vi "get Approach wfm.vi"(0 "reference in":refnum<class "Fcurve.lvclass">, 1 "Zeroed (wfms.array)":waveform(dbl)[](array[waveform]), 5 "error in (no error)":errorcluster) -> (14 "reference out":refnum<class "Fcurve.lvclass">, 15 "Zeroed (wfms.array) out":waveform(dbl)[](array[waveform]), 16 "Samples Approach":i32, 17 "Index [start,duration]":cluster{"Start":i32, "Duration":i32}, 18 "Approach":cluster{"X":dbl[], "Y":dbl[]}, 19 "error out":errorcluster)   [LabVIEW 2019, in "Fcurve.lvclass"]
uses:
  Fcurve.lvclass
  Fcurve sections.ctl
  metadata_class/Segment type--combobox.ctl
  <vilib>/Waveform/WDTOps.llb/WDT Get Waveform Subset DBL.vi
  metadata_class/metadata.lvclass
panel:
  in  "Actual seg duration":cluster{"Start":i32, "Duration":i32}[](array[cluster])
  out "index of element":i32
  out "actual duration (s)":dbl format="%0.2f"
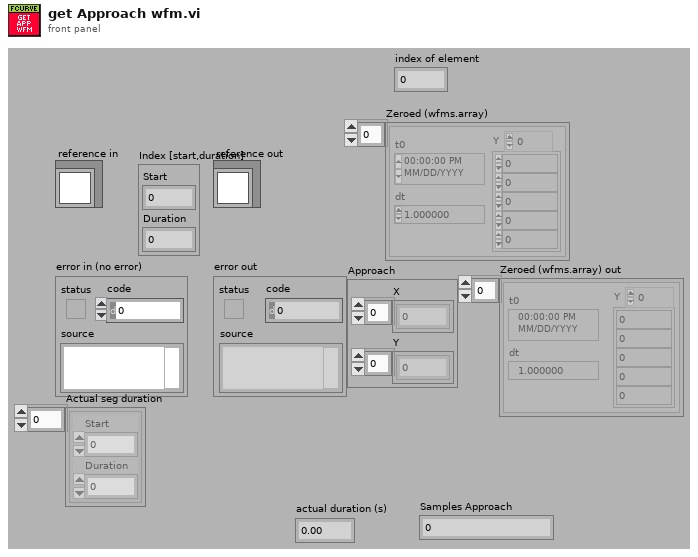
[diagram p1: front panel]
types:
  T1 = typedef "metadata.lvclass/Segment type--combobox.ctl" = string
  T2 = typedef "Fcurve.lvclass/Fcurve sections.ctl" = enum16{"Approach", "Contact", "Retract"}
  T3 = typedef "Fcurve.lvclass/ObjectAttributesRef.ctl" = refnum<data-value>
  T4 = typedef "Fcurve.lvclass/ObjectAttributes.ctl" = cluster{"MyAttribute":dbl, "Fcurve Metadata":T5, "Contact Spread of dev":dbl, "Tau Delay (ms)":dbl, "Points of contact":dbl, "Def_wfm":cluster{"Max":dbl, "Min":dbl}, "Zpos_wfm":cluster{"Max":dbl, "Min":dbl}, "Contact stat?":bool, "Real AI dt (s)":dbl, "Decimation":cluster{"App":cluster{"Dec":i32, "apply":bool}, "Con":cluster{"Dec":i32, "apply":bool}, "Ret":cluster{"Dec":i32, "apply":bool}}, "Segment def[0]":dbl, "Segment Zpos[0]":dbl, "Raw Datum":waveform(dbl)[], "Group metadata":T6, "M_data obj":refnum<class "metadata.lvclass">, "Channel name(s)":string[], "Segment fcurve data":cluster{"X":dbl[], "Y":dbl[]}[], "Segment duration":cluster{"Start":i32, "Duration":i32}[], "Segment info":T7[], "Segment durations (S)":dbl[], "Segments Maxmin":T8[]}
  T5 = typedef "Fcurve.lvclass/Metadata.ctl" = cluster{"dt (us)":dbl, "Dec Factor":dbl, "Z piezo Sensitivity (nm/V)":dbl, "K (N/m)":dbl, "Sp (V)":dbl, "Contact (ms)":dbl, "Zpos contact":dbl, "Vel_app (nm/s)":dbl, "Vel_ret (nm/s)":dbl, "deltaV (nm)":dbl, "Def_V0 (v)":dbl, "Piezo gain":dbl, "invOLS (nm/V)":dbl}
  T6 = typedef "TDMS_DataHandler.lvclass/Fcurve Meta data.ctl" = cluster{"property names":string[], "property values":variant[]}
  T7 = typedef "Fcurve.lvclass/Fcurve segments --cluster.ctl" = cluster{"type":T1, "nb points":i32, "dec factor":u32, "sampling rate (S/s)":u32}
  T8 = typedef "Fcurve.lvclass/Segment MaxMin --cluster.ctl" = cluster{"Def":cluster{"max value":dbl, "min value":dbl}, "Zpos":cluster{"max value":dbl, "min value":dbl}}
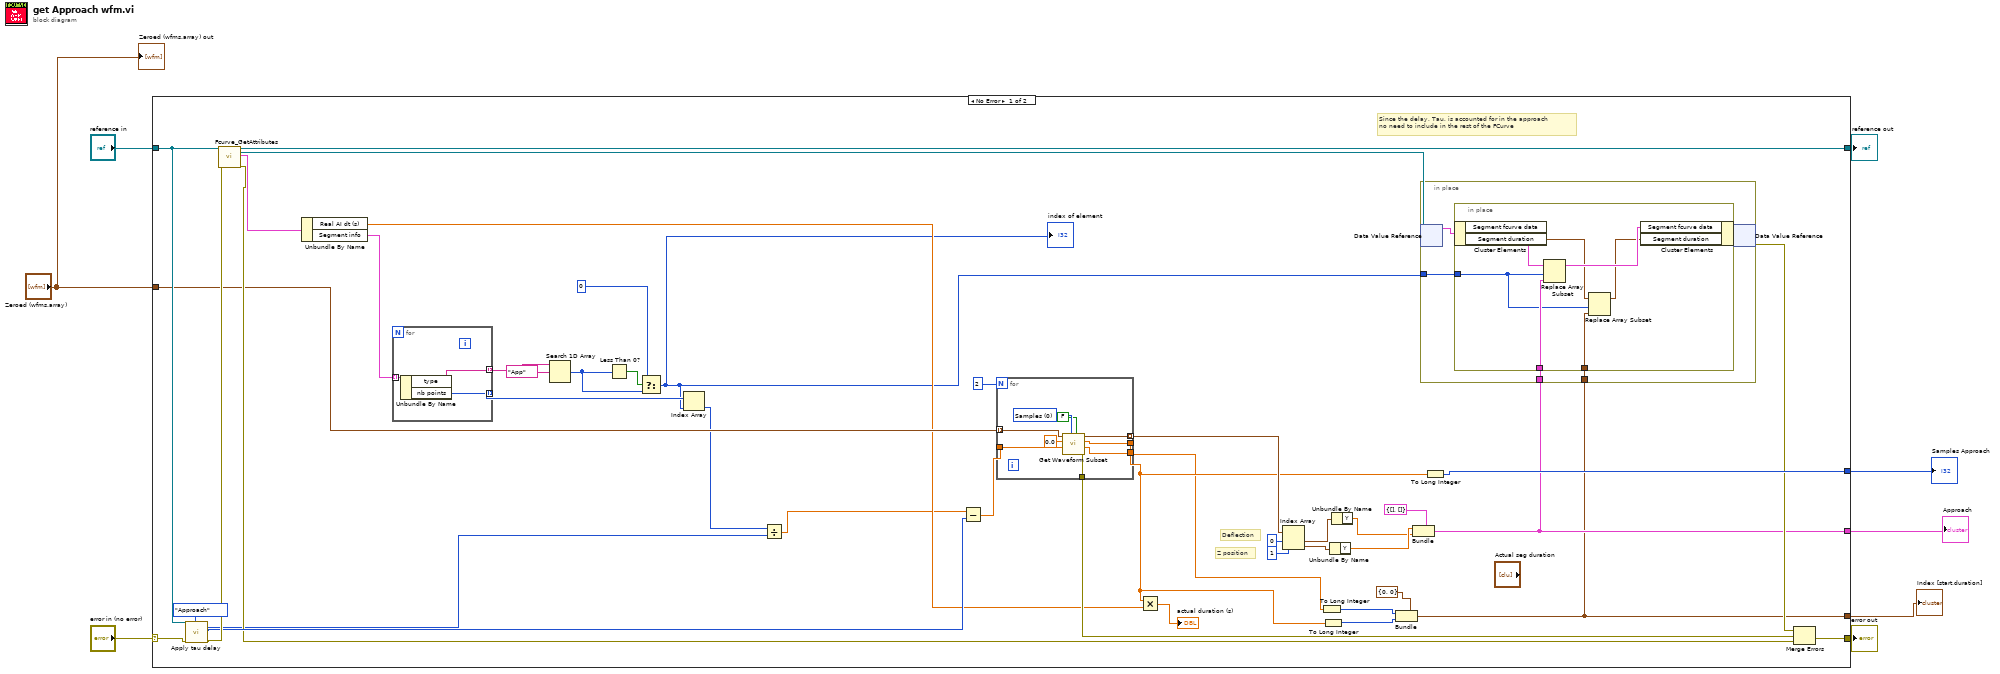
[diagram p0: block diagram]
diagram:
  n1 = case shown="No Error" "error in (no error)" {
    selector: "error in (no error)" -> [w38 w78]
    tunnel: [w52 w78] -> w7
    tunnel: [w51 w77] -> w5
    tunnel: "reference in" -> [w39 w77]
    tunnel: "Zeroed (wfms.array)" -> [w31 _]
    tunnel: [w9 _] -> w3
    tunnel: [w14 _] -> w2
    tunnel: [w30 _] -> w1
    frame No Error {
      # "Z position"
      # "Deflection"
      # "Since the delay, Tau, is accounted for in the approach\nno need to include in the rest of the FCurve"
      n2 = call "Apply tau delay.vi"("reference in"=w39, "error in (no error)"=w38, "Section"=Fcurve_sections."Approach") -> ("Dec factor"=w23:i32, "# of samples"=w36:i32, "error out"=w37:errorcluster)  [unwired: 13 in, 1 out]
      n3 = call "Fcurve_GetAttributes.vi"("reference in"=w39, "error in (no error)"=w37) -> ("reference out"=w51:refnum<class "Fcurve.lvclass">, "attributes ref"=w15:T3, "attributes"=w50:T4, "error out"=w33:errorcluster)  [unwired: 14 in]
      n4 = Unbundle By Name(w50) -> ("Real AI dt (s)"=w26:dbl, "Segment info"=w21:T7[])
      n5 = for {
        tunnel: w21 -> [w67] mode=indexing
        tunnel: [w66] -> w20 mode=indexing
        tunnel: [w65] -> w18 mode=indexing
        n6 = Unbundle By Name(w67) -> ("type"=w66:T1, "nb points"=w65:i32)
      }
      n7 = Search 1D Array(1D array=w20, element=T1 "App") -> (index of element=w12:i32)  [unwired: 1 in]
      n8 = Less Than 0?(x=w12) -> (x < 0?=w13:bool)
      n9 = Select(t=0, s=w13, f=w12) -> (s? t:f=w10:i32)
      "index of element" <- w10
      n10 = Index Array(array=w18, index=w10) -> (element=w17:i32)
      n11 = Divide(x=w17, y=w23) -> (x/y=w25:dbl)
      n12 = Subtract(x=w25, y=w36) -> (x-y=w44:dbl)
      n13 = for {
        N: 2 -> [_]
        tunnel: w44 -> [w74]
        tunnel: [w73] -> w42
        tunnel: [w72] -> w47 mode=indexing
        tunnel: w31 -> [w71] mode=indexing
        tunnel: [w69] -> w41
        tunnel: [w68] -> w32
        w76 = u16 0 items=["Samples", "Relative Time"] ("start/duration format")
        n14 = call-poly <vilib>:"Get Waveform Subset.vi"("open interval? (T)"=FALSE, "start/duration format"=w76, "duration"=w74, "start samples/time"=0.0, "waveform in"=w71) -> ("error out"=w68:errorcluster, "actual duration"=w73:dbl, "actual start samples/time"=w69:dbl, "waveform out"=w72:waveform(dbl))  [unwired: 1 in]
      }
      n15 = Multiply(x=w42, y=w26) -> (x*y=→"actual duration (s)":dbl)
      n16 = Index Array(array=w47, index #1=0 ("index"), index #2=1 ("index")) -> (element #1=w46:waveform(dbl), element #2=w45:waveform(dbl))
      n17 = To Long Integer(number=w41) -> (32bit integer=w40:i32)
      n18 = To Long Integer(number=w42) -> (32bit integer=w43:i32)
      n19 = Unbundle By Name(w45) -> ("Y"=w29:dbl[])
      n20 = Unbundle By Name(w46) -> ("Y"=w28:dbl[])
      n21 = Bundle(cluster=cluster{"Start":i32, "Duration":i32} {"Start"=0, "Duration"=0} ("Fcurve index.Contact indices"), "Start"=w40, "Duration"=w43) -> (w9:cluster{"Start":i32, "Duration":i32})
      n22 = Bundle(cluster=cluster{"X":dbl[], "Y":dbl[]} {"X"=[], "Y"=[]} ("Fcurve.Approach"), "X"=w29, "Y"=w28) -> (w14:cluster{"X":dbl[], "Y":dbl[]})
      n23 = in-place {
        in-place-border: w14 -> [w55]
        in-place-border: w10 -> [w54]
        in-place-border: w9 -> [w53]
        n24 = in-place-dvr #1(w15) -> (w56:T4)  [unwired: 1 out]
        n25 = in-place {
          in-place-border: w55 -> [w62]
          in-place-border: w54 -> [w58]
          in-place-border: w53 -> [w59]
          n26 = in-place-cluster #2(w56) -> ("Segment fcurve data"=w64:cluster{"X":dbl[], "Y":dbl[]}[], "Segment duration"=w61:cluster{"Start":i32, "Duration":i32}[])
          n27 = Replace Array Subset(array=w64, new element=w62, index=w58) -> (w63:cluster{"X":dbl[], "Y":dbl[]}[])
          n28 = Replace Array Subset(array=w61, new element=w59, index=w58) -> (w60:cluster{"Start":i32, "Duration":i32}[])
          n29 = in-place-cluster #2("Segment fcurve data"=w63, "Segment duration"=w60) -> (w57:T4)
        }
        n30 = in-place-dvr #1(w57) -> (w16:errorcluster)  [unwired: 1 out]
      }
      n31 = To Long Integer(number=w42) -> (32bit integer=w30:i32)
      n32 = Merge Errors(w16, w32, w33) -> (w52:errorcluster)
    }
    frame Error {
    }
  }
  "error out" <- w7
  "reference out" <- w5
  "Index [start,duration]" <- w3
  "Approach" <- w2
  "Samples Approach" <- w1
  "Zeroed (wfms.array) out" <- "Zeroed (wfms.array)"
